vi "LoadIntoSubPanel.vi"(8 "error in (no error)":errorcluster, 10 "VI Refnum":refnum<vi>, 11 "CameraTesting in":refnum<class "CameraTesting.lvclass">) -> (0 "error out":errorcluster, 3 "CameraTesting out":refnum<class "CameraTesting.lvclass">)   [LabVIEW 2020, in "CameraTesting.lvlib" / "CameraTesting.lvclass"]
uses:
  CameraTesting.lvclass
  CameraTesting.lvclass/CameraTesting.ctl
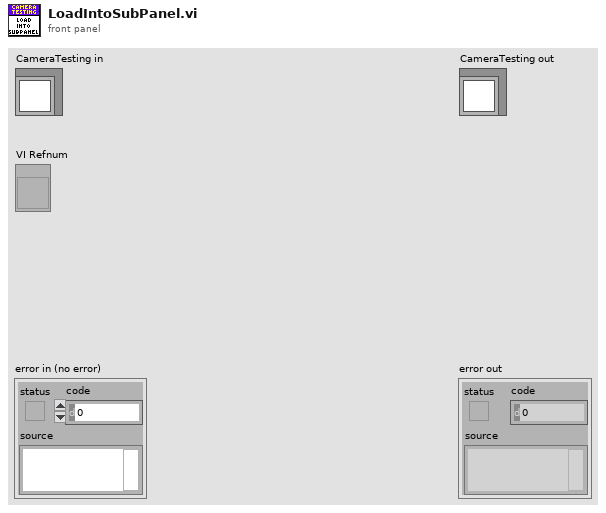
[diagram p1: front panel]
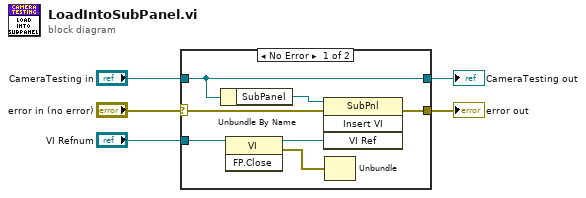
[diagram p0: block diagram]
diagram:
  n1 = case shown="No Error" "error in (no error)" {
    selector: "error in (no error)" -> [w8 w14]
    tunnel: "CameraTesting in" -> [w9 w13]
    tunnel: "VI Refnum" -> [w12 _]
    tunnel: [w7 w14] -> w2
    tunnel: [w9 w13] -> w1
    frame No Error {
      n2 = Unbundle By Name(w9) -> ("SubPanel"=w11:refnum<vi>)
      n3 = invoke class="VI" method="FP.Close"(reference=w12) -> (reference out=w10:refnum<vi>, error out=w6:errorcluster)  [unwired: 2 in, 1 out]
      n4 = invoke class="SubPnl" method="Insert VI"(reference=w11, error in=w8, "VI Ref"=w10) -> (error out=w7:errorcluster)  [unwired: 1 in, 3 out]
      n5 = Unbundle(w6) -> ()  [unwired: 3 out]
    }
    frame Error {
    }
  }
  "error out" <- w2
  "CameraTesting out" <- w1
